vi "initial stuff.vi"(1 "select file":path) -> (0 "Map Data":T1)   [LabVIEW 2009]
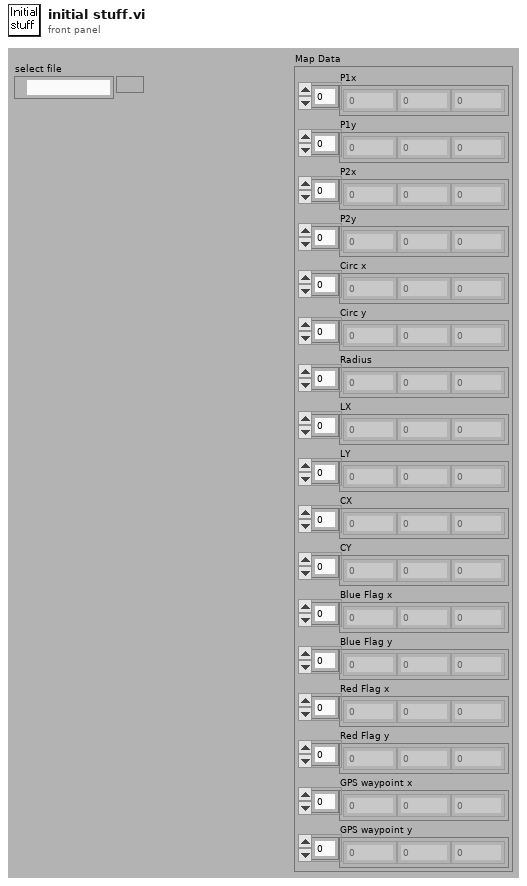
[diagram p1: front panel]
types:
  T1 = cluster{"P1x":dbl[], "P1y":dbl[], "P2x":dbl[], "P2y":dbl[], "Circ x":dbl[], "Circ y":dbl[], "Radius":dbl[], "LX":dbl[], "LY":dbl[], "CX":dbl[], "CY":dbl[], "Blue Flag x":dbl[], "Blue Flag y":dbl[], "Red Flag x":dbl[], "Red Flag y":dbl[], "GPS waypoint x":dbl[], "GPS waypoint y":dbl[]}
  T2 = cluster{"P1x":dbl[], "P1y":dbl[], "P2x":dbl[], "P2y":dbl[], "Circ x":dbl[], "Circ y":dbl[], "Radius":dbl[], "Blue Flag x":dbl[], "Blue Flag y":dbl[], "Red Flag x":dbl[], "Red Flag y":dbl[], "GPS waypoint x":dbl[], "GPS waypoint y":dbl[]}
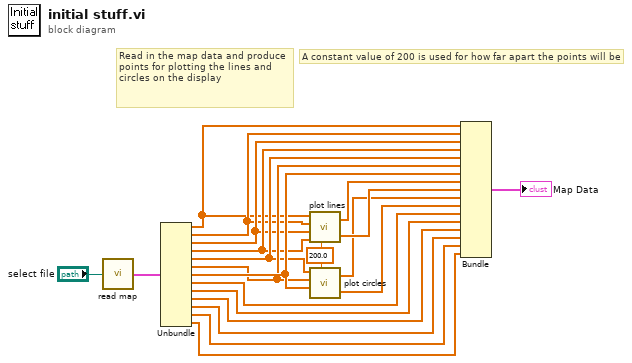
[diagram p0: block diagram]
diagram:
  w10 = 200.0 ("dL")
  # "Read in the map data and produce points for plotting the lines and circles on the display"
  # "A constant value of 200 is used for how far apart the points will be"
  n1 = call "read map.vi"("select file"="select file") -> ("Map Data"=w9:T2)
  n2 = Unbundle(w9) -> ("P1x"=w11:dbl[], "P1y"=w12:dbl[], "P2x"=w13:dbl[], "P2y"=w14:dbl[], "Circ x"=w15:dbl[], "Circ y"=w16:dbl[], "Radius"=w17:dbl[], "Blue Flag x"=w7:dbl[], "Blue Flag y"=w6:dbl[], "Red Flag x"=w5:dbl[], "Red Flag y"=w4:dbl[], "GPS waypoint x"=w3:dbl[], "GPS waypoint y"=w2:dbl[])
  n3 = call "plot lines.vi"("P1x"=w11, "P1y"=w12, "P2x"=w13, "P2y"=w14, "dL"=w10) -> ("LX"=w20:dbl[], "LY"=w21:dbl[])
  n4 = call "plot circles.vi"("dL"=w10, "Radius"=w17, "Circle y"=w16, "Circle x"=w15) -> ("CY"=w19:dbl[], "CX"=w18:dbl[])
  n5 = Bundle("P1x"=w11, "P1y"=w12, "P2x"=w13, "P2y"=w14, "Circ x"=w15, "Circ y"=w16, "Radius"=w17, "LX"=w20, "LY"=w21, "CX"=w18, "CY"=w19, "Blue Flag x"=w7, "Blue Flag y"=w6, "Red Flag x"=w5, "Red Flag y"=w4, "GPS waypoint x"=w3, "GPS waypoint y"=w2) -> (→"Map Data":T1)  [unwired: 1 in]
